vi "Avg Values 2.vi"(0 "Digital in":refnum<vi>, 1 "Numeric 8":dbl, 2 "Numeric 4":dbl, 3 "Numeric 9":dbl, 4 "Numeric 3":dbl, 6 "Numeric 5":dbl, 7 "Numeric in":dbl, 8 "reference in":refnum<vi>, 9 "Numeric 12":dbl, 10 "Numeric 6":dbl, 11 "Numeric 11":dbl, 13 "Numeric 10":dbl) -> (14 "Numeric 7":dbl, 15 "Numeric out":dbl)   [LabVIEW 2014]
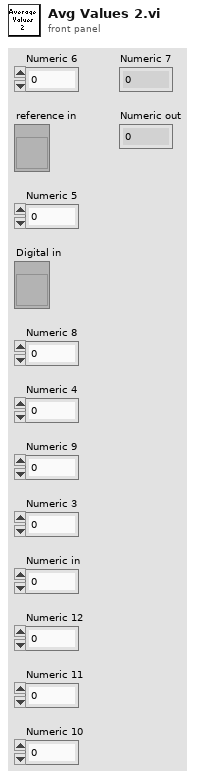
[diagram p1: front panel]
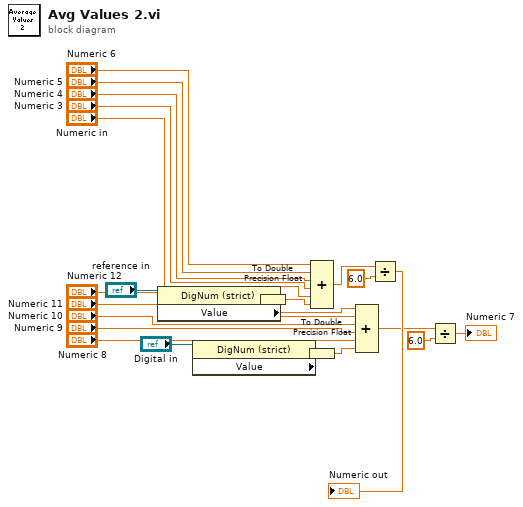
[diagram p0: block diagram]
diagram:
  n1 = property class="DigNum (strict)"(reference="reference in") -> ("Value"=w4:fxp<+,64,16>)  [unwired: 1 in, 2 out]
  n2 = property class="DigNum (strict)"(reference="Digital in") -> ("Value"=w3:fxp<+,64,16>)  [unwired: 1 in, 2 out]
  n3 = To Double Precision Float(number=w4) -> (double precision float=w16:dbl)
  n4 = To Double Precision Float(number=w3) -> (double precision float=w12:dbl)
  n5 = Compound Arithmetic op=ADD("Numeric 6", "Numeric 5", "Numeric 4", "Numeric 3", "Numeric in", w16) -> (w14:dbl)
  n6 = Compound Arithmetic op=ADD("Numeric 12", "Numeric 11", "Numeric 10", "Numeric 9", "Numeric 8", w12) -> (w6:dbl)
  n7 = Divide(x=w14, y=6.0) -> (x/y=→"Numeric out":dbl)
  n8 = Divide(x=w6, y=6.0) -> (x/y=→"Numeric 7":dbl)
